vi "TICK-TACK.vi"(10 "calkowity okres":u64=2, 11 "czas za³aczenia":u64=1000) -> (3 "Timeout":bool)   [LabVIEW 2015]
panel:
  in  "Timeout Period 2":u64=1000
  out "floor(x/y)":u64
  out "x-y*floor(x/y)":u64
  out "Elapsed Time":u64
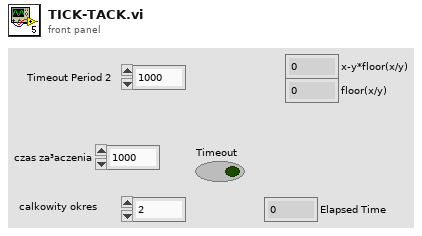
[diagram p1: front panel]
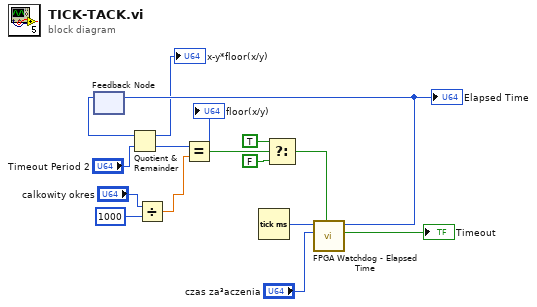
[diagram p0: block diagram]
diagram:
  n1 = feedback #1() -> (w10:u64)  [unwired: 1 in]
  n2 = Quotient & Remainder(x=w10, y="Timeout Period 2") -> (x-y*floor(x/y)=→"x-y*floor(x/y)":u64, floor(x/y)=w14:u64)
  "floor(x/y)" <- w14
  n3 = Divide(x="calkowity okres", y=u64 1000) -> (x/y=w2:dbl)
  n4 = Equal?(x=w14, y=w2) -> (x = y?=w15:bool)
  n5 = Tick Count (ms)() -> (millisecond timer value=w5:u32)
  n6 = Select(t=TRUE, s=w15, f=FALSE) -> (s? t:f=w9:bool)
  n7 = call "FPGA Watchdog - Elapsed Time.vi"("Reset"=w9, "Timeout Period"="czas za³aczenia", "Current Time"=w5) -> ("Timeout"=→"Timeout":bool, "Elapsed Time"=w8:u64)  [unwired: 7 in]
  "Elapsed Time" <- w8
  n8 = feedback-in #1(w8) -> ()
